vi "ConfigMultifileWrite.vi"(10 "Reference":T1) -> (2 "Data Valid":bool)   [LabVIEW 2020]
uses:
  <vilib>/express/express shared/propPageData.ctl
panel:
  in  "max_elapsed_seconds":i32
  in  "Time":i32 min=0 max=86399 step=60 format="%<%H:%M>t"
  in  "Hours":i32 min=0 max=999
  in  "Help":bool
  in  "Ok":bool
  in  "Cancel":bool
  in  "overwrite_mode_multi":i32
  in  "new_file_mode":i32
  in  "Use next available filename":bool
  in  "Overwrite file":bool
  in  "Rename existing file":bool
  out "Filename preview":string
  in  "Both":bool
  in  "fixed_width":bool=TRUE
  in  "Width":i32=2 min=1 max=9
  in  "Date and time":bool=TRUE
  in  "Sequential numbers":bool
  in  "Samples":i32=1 min=1
  in  "Segments":i32=1 min=1
  in  "new_file_samples":bool
  in  "new_file_iter":bool
  in  "new_file_daily":bool
  in  "Minutes":i32 min=0 max=59
  in  "new_file_elaps_time":bool
  in  "KB":i32=100
  in  "new_file_size":bool=TRUE
  in  "file_path":path=path "testdata_.txt"
  in  "time_format_string":string="%Y-%m-%d"
  # "Filename Suffix"
  # "File Termination"
  # "Condition for starting a new file"
  # "Existing Files"
  # "Action to take if the file already exists"
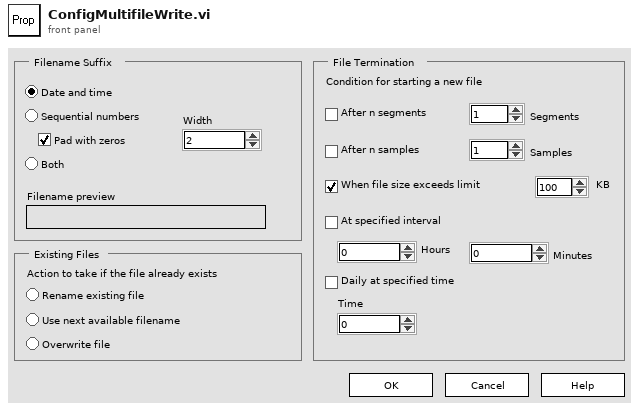
[diagram p1: front panel]
types:
  T1 = typedef "propPageData.ctl" = cluster{"InstanceCtlRefs":refnum<vi>[], "ConfigDlgCtlRefs":refnum<vi>[], "Control Data":cluster{"Ctl Type":u16, "Instance Ctl Label":string, "Config Dialog Ctl Label":string}[], "viref Instance":refnum<vi>, "Types":i32[], "Config DialogVI":refnum<vi>}
  T2 = enum8{"Enabled", "Disabled", "Disabled and Grayed Out"}
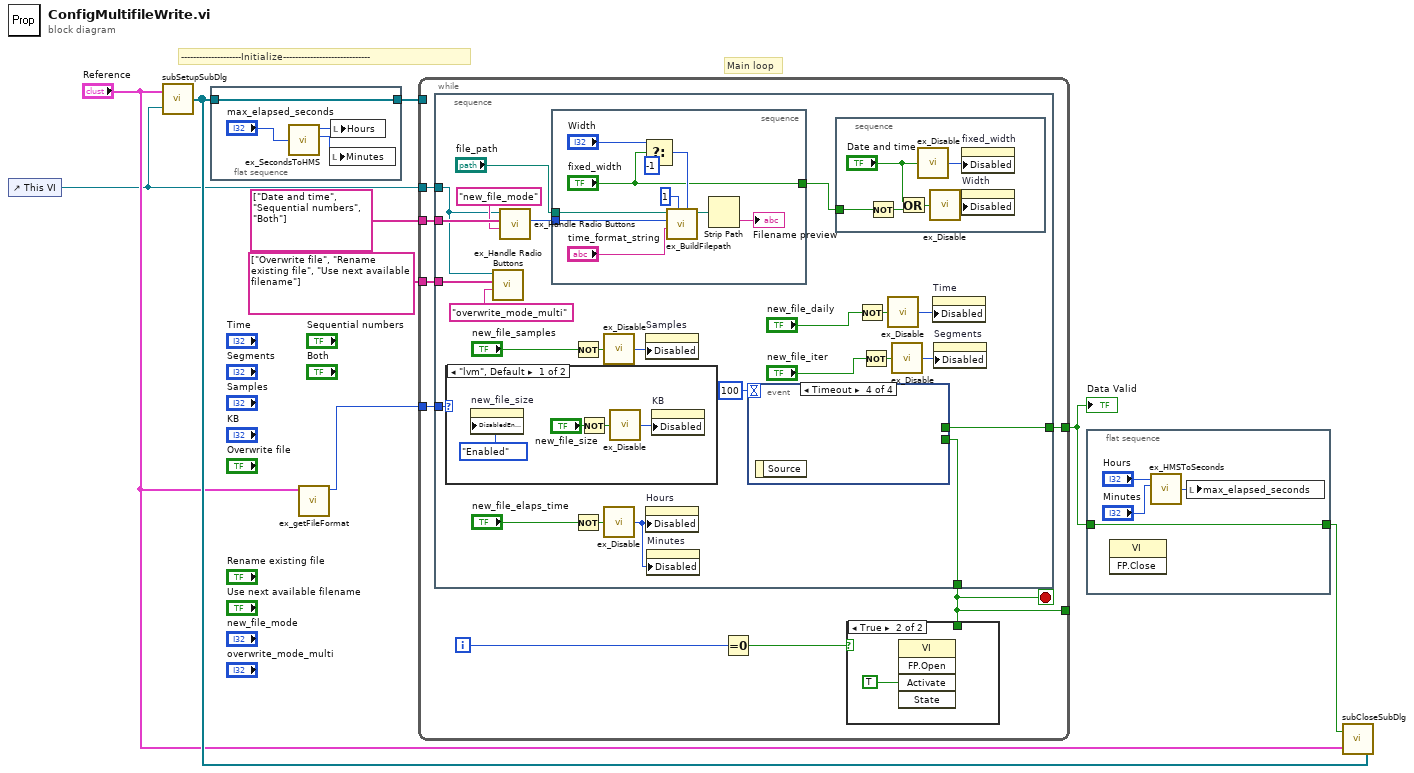
[diagram p0: block diagram]
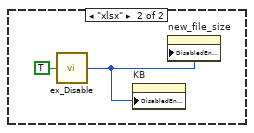
[diagram p3: hidden frame]
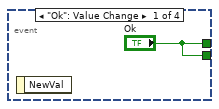
[diagram p4: hidden frame]
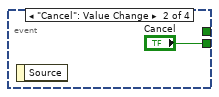
[diagram p5: hidden frame]
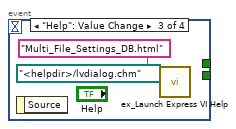
[diagram p6: hidden frame]
diagram:
  # "--------------------Initialize-----------------------------"
  # "Main loop"
  n1 = control-ref of="This VI"() -> (w1:refnum<vi>)
  n2 = call <vilib>:"subSetupSubDlg.vi"("viref subdlg"=w1, "Reference"="Reference") -> ("subDlgRefs"=w7:refnum<vi>[])
  n3 = flat-sequence {
    tunnel: w7 -> [w11]
    tunnel: [w11] -> w6
    frame #0 {
      n4 = call <vilib>:"ex_SecondsToHMS.vi"("seconds"="max_elapsed_seconds") -> ("hours"=w12:i32, "minutes"=w10:i32)  [unwired: 2 out]
      n5 = local write "Minutes"(w10) -> ()
      n6 = local write "Hours"(w12) -> ()
    }
  }
  n7 = call <vilib>:"ex_getFileFormat.vi"("Reference"="Reference") -> ("storage_format"=w2:enum32{"lvm", "tdm", "tdms", "xlsx"})  [unwired: 10 in]
  n8 = while {
    tunnel: [w21] -> w5
    tunnel: w1 -> [w19]
    tunnel: string[] ["Date and time", "Sequential numbers", "Both"] ("Radio Buttons") -> [w20]
    tunnel: string[] ["Overwrite file", "Rename existing file", "Use next available filename"] ("Radio Buttons") -> [w18]
    tunnel: w6 -> [_]
    tunnel: [w15] -> _
    tunnel: w2 -> [w14]
    i -> [w16]
    stop <- w15 stop-if-true
    n9 = stacked-sequence {
      tunnel: [w30] -> w21
      tunnel: w20 -> [w46]
      tunnel: w19 -> [w34]
      tunnel: [w29] -> w15
      tunnel: w18 -> [w36]
      tunnel: w14 -> [w23]
      frame #0 {
        n10 = case shown="\"lvm\", Default" w23 {
          frame "lvm", Default {
            n11 = property on="new_file_size" class="Bool (strict)"("DisabledEnum"=T2."Enabled" ("Disabled")) -> ()  [unwired: 2 in, 2 out]
            n12 = Not(x="new_file_size") -> (.not. x?=w48:bool)
            n13 = call <vilib>:"ex_Disable.vi"("Disable?"=w48) -> ("Disabled value"=w49:u8)
            n14 = property on="KB" class="DigNum (strict)"("Disabled"=w49) -> ()  [unwired: 2 in, 2 out]
          }
          frame "xlsx" {
            n15 = call <vilib>:"ex_Disable.vi"("Disable?"=TRUE) -> ("Disabled value"=w51:u8)
            n16 = property on="KB" class="DigNum (strict)"("DisabledEnum"=w51) -> ()  [unwired: 2 in, 2 out]
            n17 = property on="new_file_size" class="Bool (strict)"("DisabledEnum"=w51) -> ()  [unwired: 2 in, 2 out]
          }
        }
        n18 = call <vilib>:"ex_Handle Radio Buttons.vi"("Numeric Control"="overwrite_mode_multi", "Radio Buttons"=w36, "VI refnum"=w34) -> ()  [unwired: 4 in, 5 out]
        n19 = call <vilib>:"ex_Handle Radio Buttons.vi"("Numeric Control"="new_file_mode", "Radio Buttons"=w46, "VI refnum"=w34) -> ("Selected Button"=w33:u32)  [unwired: 4 in, 4 out]
        n20 = stacked-sequence {
          tunnel: w33 -> [w72]
          tunnel: "file_path" -> [w68]
          tunnel: ["fixed_width"] -> w38
          frame #0 {
            n21 = Select(t="Width", s="fixed_width", f=-1 ("serno_digits")) -> (s? t:f=w70:i32)
            n22 = call <vilib>:"ex_BuildFilepath.vi"("serial digits"=w70, "serial num"=1, "time format string"="time_format_string", "naming mode"=w72, "name base"=w68) -> ("built name"=w67:path)  [unwired: 1 in, 5 out]
            n23 = Strip Path(path=w67) -> (name=→"Filename preview":string)  [unwired: 1 out]
          }
        }
        n24 = Not(x="new_file_samples") -> (.not. x?=w40:bool)
        n25 = Not(x="new_file_elaps_time") -> (.not. x?=w45:bool)
        n26 = call <vilib>:"ex_Disable.vi"("Disable?"=w40) -> ("Disabled value"=w39:u8)
        n27 = call <vilib>:"ex_Disable.vi"("Disable?"=w45) -> ("Disabled value"=w44:u8)
        n28 = property on="Samples" class="DigNum (strict)"("Disabled"=w39) -> ()  [unwired: 2 in, 2 out]
        n29 = property on="Hours" class="DigNum (strict)"("Disabled"=w44) -> ()  [unwired: 2 in, 2 out]
        n30 = property on="Minutes" class="DigNum (strict)"("Disabled"=w44) -> ()  [unwired: 2 in, 2 out]
        n31 = event shown="[3] Timeout" {
          selector: _ -> [_ _ _ _]
          dyn-events: _ -> [_ _ _ _]
          timeout: 100 -> [_ _ _ _]
          tunnel: ["Ok" _ _ _] -> w30
          tunnel: ["Ok" "Cancel" _ _] -> w29
          event "Ok": Value Change {
            n32 = event-data() -> ()  [unwired: 2 out]
          }
          event "Cancel": Value Change {
            n33 = event-data() -> ()  [unwired: 2 out]
          }
          event "Help": Value Change {
            n34 = event-data() -> ()  [unwired: 2 out]
            n35 = call <vilib>:"ex_Launch Express VI Help.vi"("Help File Path"=path "<helpdir>/lvdialog.chm", "Keyword/HTML File"="Multi_File_Settings_DB.html" ("Help string to search for")) -> ()  [unwired: 1 in, 5 out]
          }
          event Timeout {
            n36 = event-data() -> ()  [unwired: 2 out]
          }
        }
        n37 = stacked-sequence {
          tunnel: w38 -> [w62]
          frame #0 {
            n38 = Not(x=w62) -> (.not. x?=w58:bool)
            n39 = Or(x="Date and time", y=w58) -> (x .or. y?=w59:bool)
            n40 = call <vilib>:"ex_Disable.vi"("Disable?"="Date and time") -> ("Disabled value"=w61:u8)
            n41 = call <vilib>:"ex_Disable.vi"("Disable?"=w59) -> ("Disabled value"=w60:u8)
            n42 = property on="fixed_width" class="Bool (strict)"("Disabled"=w61) -> ()  [unwired: 2 in, 2 out]
            n43 = property on="Width" class="DigNum (strict)"("Disabled"=w60) -> ()  [unwired: 2 in, 2 out]
          }
        }
        n44 = Not(x="new_file_daily") -> (.not. x?=w43:bool)
        n45 = Not(x="new_file_iter") -> (.not. x?=w42:bool)
        n46 = call <vilib>:"ex_Disable.vi"("Disable?"=w43) -> ("Disabled value"=w31:u8)
        n47 = call <vilib>:"ex_Disable.vi"("Disable?"=w42) -> ("Disabled value"=w41:u8)
        n48 = property on="Time" class="DigNum (strict)"("Disabled"=w31) -> ()  [unwired: 2 in, 2 out]
        n49 = property on="Segments" class="DigNum (strict)"("Disabled"=w41) -> ()  [unwired: 2 in, 2 out]
      }
    }
    n50 = Equal To 0?(x=w16) -> (x = 0?=w17:bool)
    n51 = case shown="True" w17 {
      tunnel: w15 -> [_ _]
      frame False {
      }
      frame True {
        n52 = invoke class="VI" method="FP.Open"("Activate"=TRUE ("Front Panel Window:Open")) -> ()  [unwired: 4 in, 5 out]
      }
    }
  }
  "Data Valid" <- w5
  n53 = flat-sequence {
    tunnel: w5 -> [w76]
    tunnel: [w76] -> w4
    frame #0 {
      n54 = invoke class="VI" method="FP.Close"() -> ()  [unwired: 3 in, 3 out]
      n55 = call <vilib>:"ex_HMSToSeconds.vi"("minutes"="Minutes", "hours"="Hours") -> ("seconds"=w73:i32)  [unwired: 1 in, 1 out]
      n56 = local write "max_elapsed_seconds"(w73) -> ()
    }
  }
  n57 = call <vilib>:"subCloseSubDlg.vi"("subDlgRefs"=w7, "Reference"="Reference", "OK Pressed"=w4) -> ()
